vi "Untitled 5.vi"() -> ()   [LabVIEW 2015]
panel:
  out "Sub":string[](array[string])
  out "Main":string[](array[string])
  out "共同":string[](array[string])
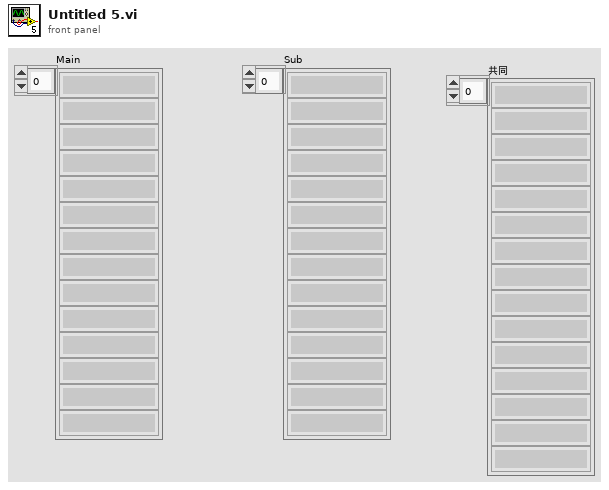
[diagram p1: front panel]
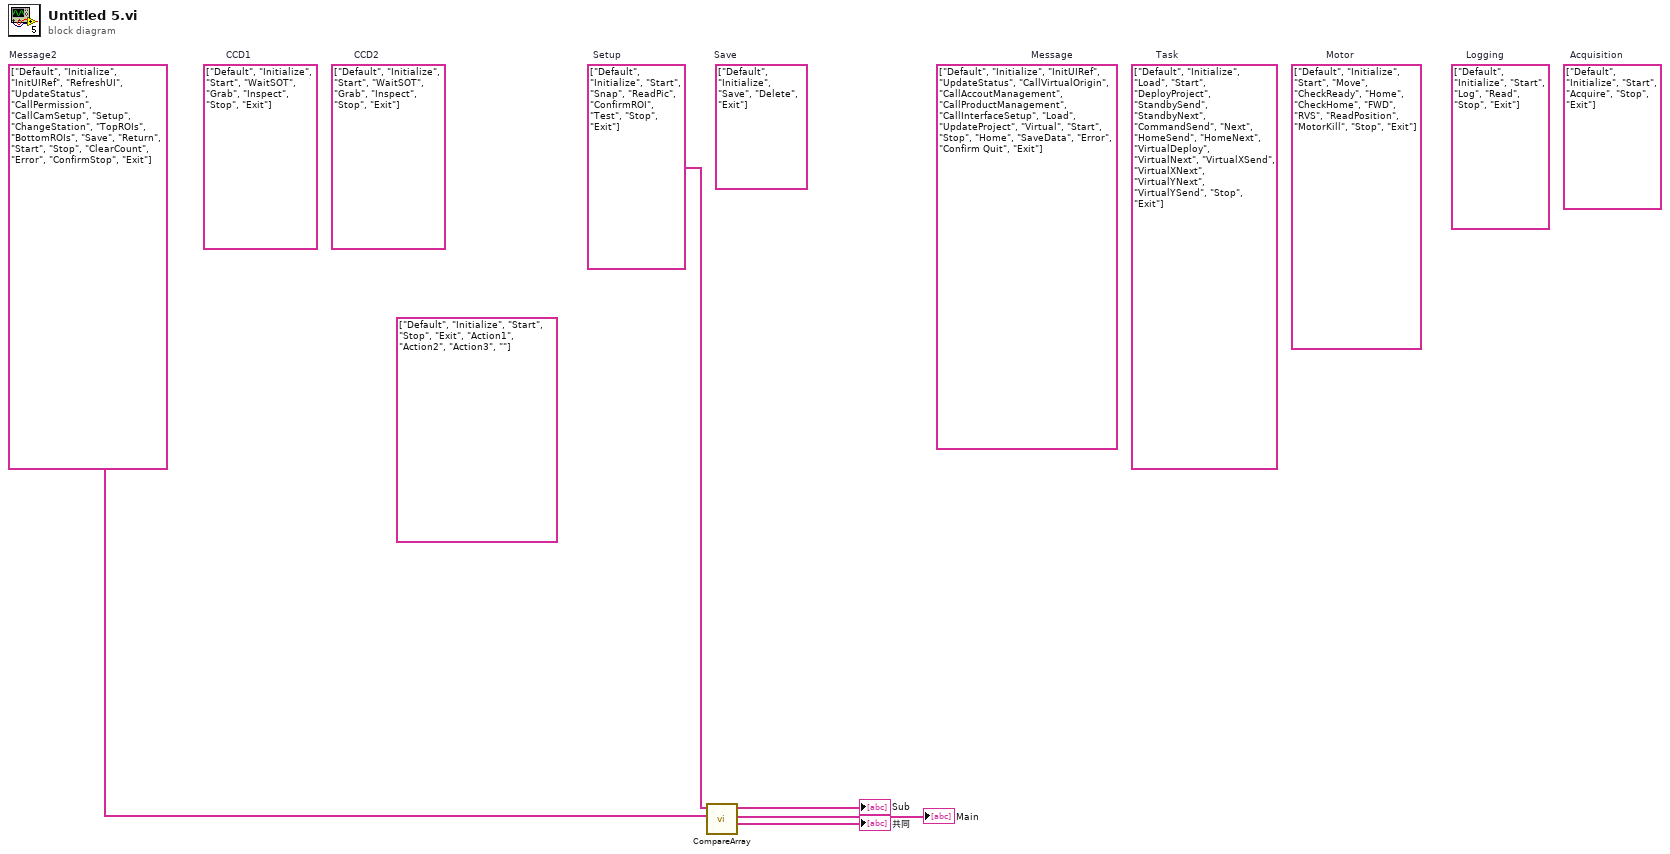
[diagram p0: block diagram]
diagram:
  (unwired) string[] ["Default", "Initialize", "Start", "Stop", "Exit", "Action1", "Action2", "Action3", ""] ("Array")
  (unwired) string[] ["Default", "Initialize", "Save", "Delete", "Exit"]  # Save
  (unwired) string[] ["Default", "Initialize", "Start", "WaitSOT", "Grab", "Inspect", "Stop", "Exit"]  # CCD2
  w4 = string[] ["Default", "Initialize", "Start", "Snap", "ReadPic", "ConfirmROI", "Test", "Stop", "Exit"]  # Setup
  (unwired) string[] ["Default", "Initialize", "Start", "WaitSOT", "Grab", "Inspect", "Stop", "Exit"]  # CCD1
  w5 = string[] ["Default", "Initialize", "InitUIRef", "RefreshUI", "UpdateStatus", "CallPermission", "CallCamSetup", "Setup", "ChangeStation", "TopROIs", "BottomROIs", "Save", "Return", "Start", "Stop", "ClearCount", "Error", "ConfirmStop", "Exit"]  # Message2
  (unwired) string[] ["Default", "Initialize", "Start", "Acquire", "Stop", "Exit"]  # Acquisition
  (unwired) string[] ["Default", "Initialize", "Start", "Log", "Read", "Stop", "Exit"]  # Logging
  (unwired) string[] ["Default", "Initialize", "Start", "Move", "CheckReady", "Home", "CheckHome", "FWD", "RVS", "ReadPosition", "MotorKill", "Stop", "Exit"]  # Motor
  (unwired) string[] ["Default", "Initialize", "Load", "Start", "DeployProject", "StandbySend", "StandbyNext", "CommandSend", "Next", "HomeSend", "HomeNext", "VirtualDeploy", "VirtualNext", "VirtualXSend", "VirtualXNext", "VirtualYNext", "VirtualYSend", "Stop", "Exit"]  # Task
  (unwired) string[] ["Default", "Initialize", "InitUIRef", "UpdateStatus", "CallVirtualOrigin", "CallAccoutManagement", "CallProductManagement", "CallInterfaceSetup", "Load", "UpdateProject", "Virtual", "Start", "Stop", "Home", "SaveData", "Error", "Confirm Quit", "Exit"]  # Message
  n1 = call "CompareArray.vi"("Array2"=w5, "Array1"=w4) -> ("共同"=→"共同":string[], "Main"=→"Main":string[], "Sub"=→"Sub":string[])  [unwired: 7 in]
